vi "Send Message Immediate.vi"(8 "error in":errorcluster, 10 "IMessage":refnum<class "IMessage.lvclass">, 11 "Simulated CANopen Node in":refnum<class "Simulated CANopen Node.lvclass">) -> (0 "error out":errorcluster, 3 "Simulated CANopen Node out":refnum<class "Simulated CANopen Node.lvclass">)   [LabVIEW 2020, in "Simulated CANopen Node.lvclass"]
uses:
  Simulated CANopen Node.lvclass
  HAL/Source/Interfaces/IMessage/IMessage.lvclass
  Simulated CANopen Node.lvclass/Simulated CANopen Node.ctl
  HAL/Source/Messages/CAN CC Frame/CAN CC Frame.lvclass
  fe5fc66b-27c7-4b70-867a-ed015ee1e4a2.vi
  eee18dc1-6225-4693-ac9d-30609a8fa5c9.vi
  17ac248f-ac84-4826-aeec-a58701ccab40.vi
  98e92c24-c08f-4278-8538-098933e240cd.vi
  56a45396-c398-4984-a56f-735f0d2926b6.vi
  7e0a11d8-4694-4177-9e19-67e5199e02f7.vi
  5fa304e1-3e3d-4d0b-887e-d9a5c5a4f673.vi
  7c59c303-af64-4ebe-8db4-2588cd71c9a9.vi
  1c0038d2-8b70-42b8-b8fb-ff38a0514d58.vi
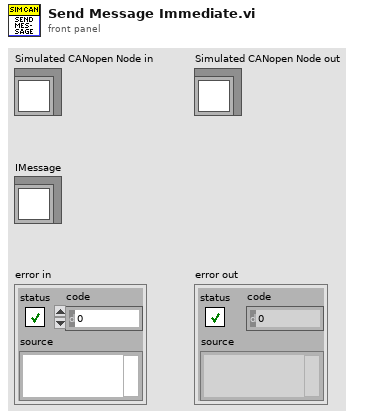
[diagram p1: front panel]
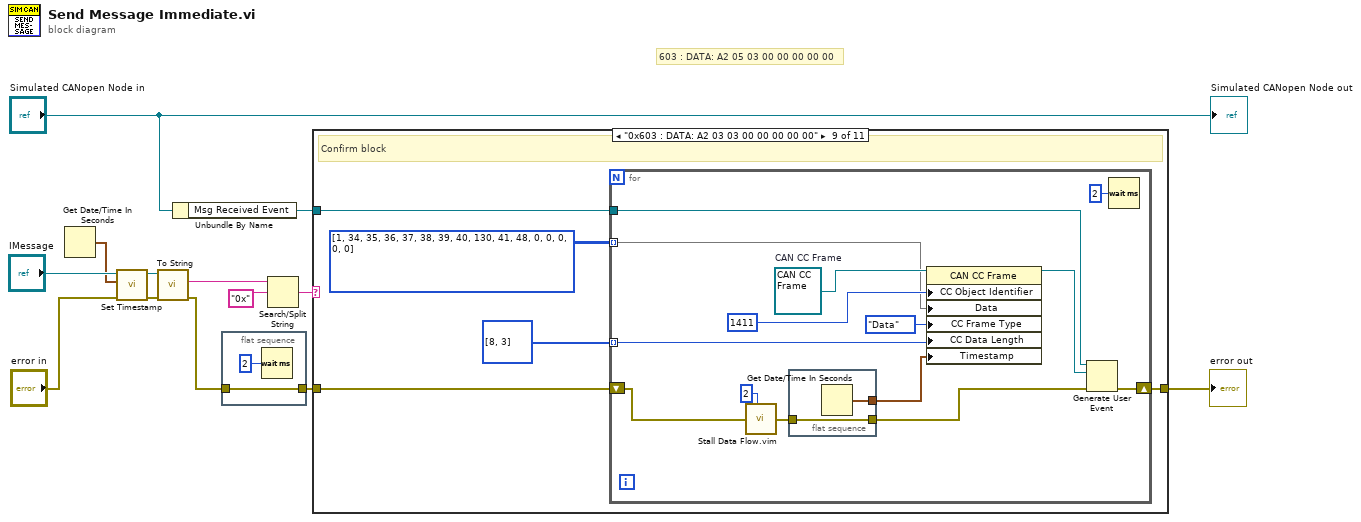
[diagram p0: block diagram]
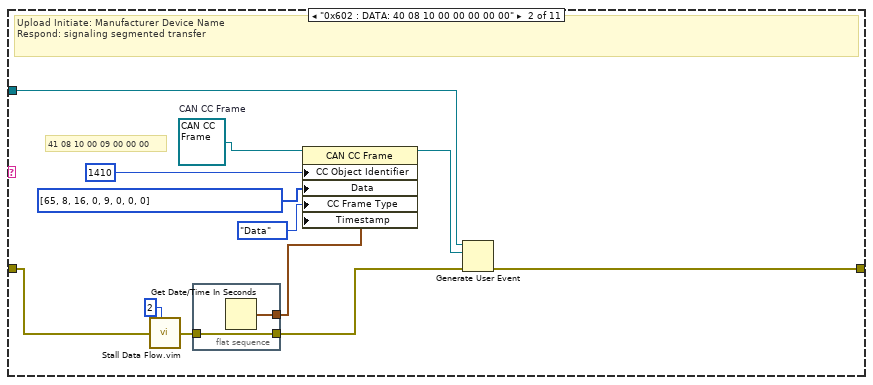
[diagram p3: hidden frame]
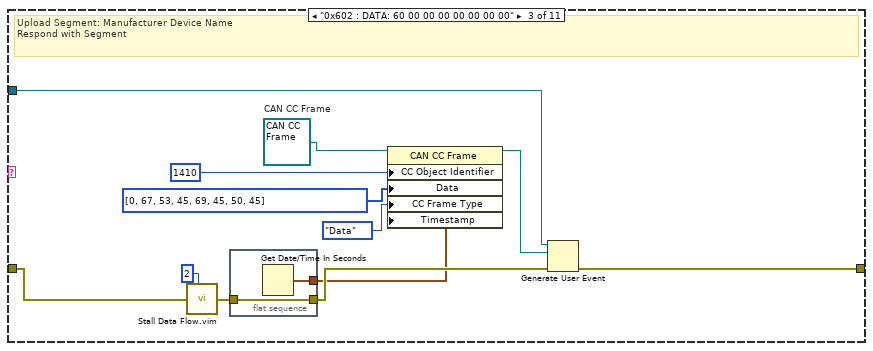
[diagram p4: hidden frame]
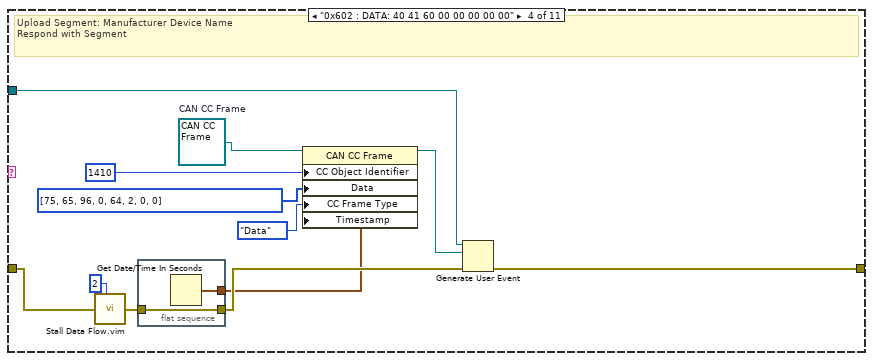
[diagram p5: hidden frame]
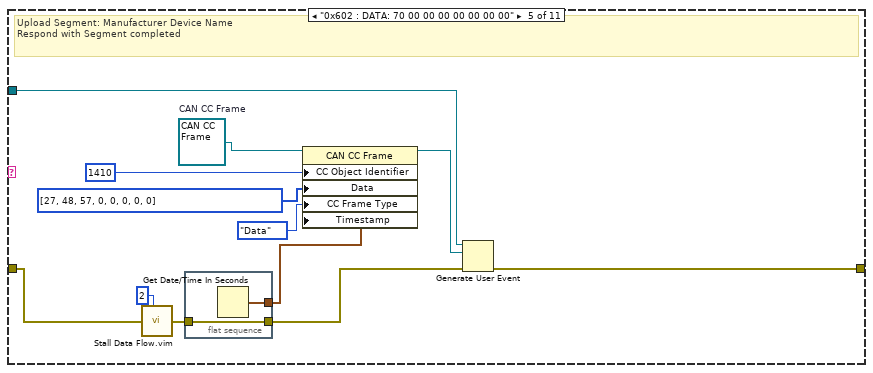
[diagram p6: hidden frame]
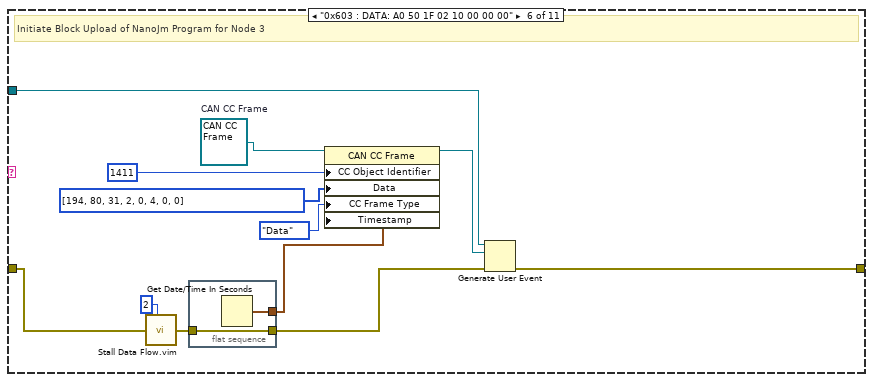
[diagram p7: hidden frame]
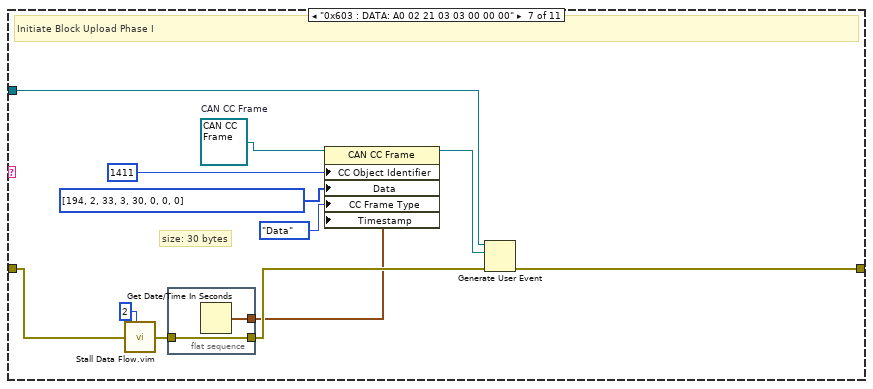
[diagram p8: hidden frame]
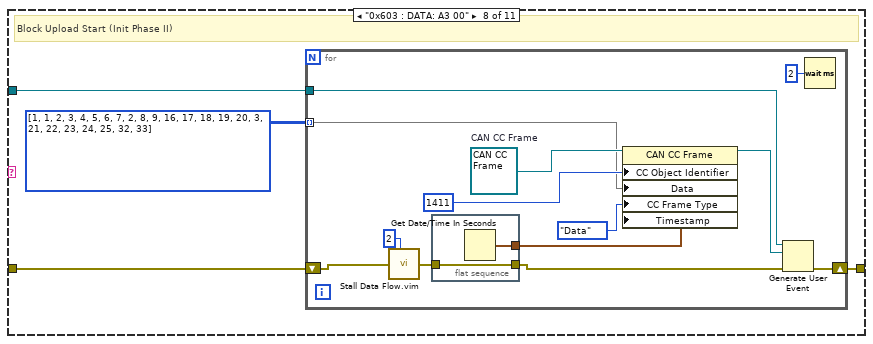
[diagram p9: hidden frame]
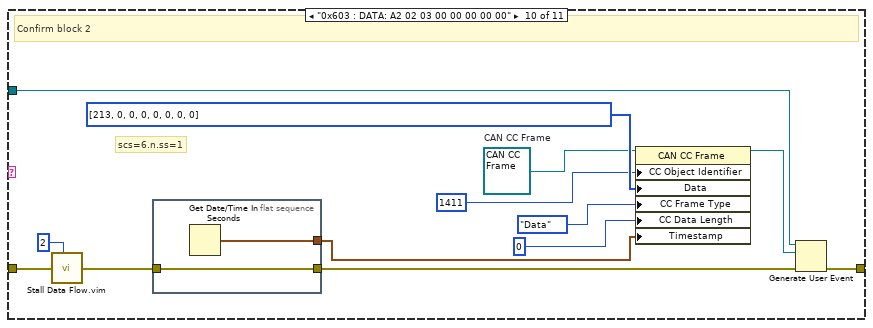
[diagram p10: hidden frame]
diagram:
  # "603 : DATA: A2 05 03 00 00 00 00 00"
  n1 = Get Date/Time In Seconds() -> (seconds since 1Jan1904=w1:timestamp)
  n2 = call-dynamic "Set Timestamp.vi"("error in"="error in", "Time Stamp"=w1, "IMessage in"="IMessage") -> ("error out"=w4:errorcluster, "IMessage out"=w2:refnum<class "IMessage.lvclass">)  [unwired: 7 in]
  n3 = call-dynamic "To String.vi"("error in"=w4, "IMessage in"=w2) -> ("error out"=w6:errorcluster, "Stringified"=w11:string)  [unwired: 7 in, 1 out]
  n4 = Unbundle By Name("Simulated CANopen Node in") -> ("Msg Received Event"=w9:refnum<user-event>)
  n5 = flat-sequence {
    tunnel: w6 -> [w14]
    tunnel: [w14] -> w5
    frame #0 {
      n6 = Wait (ms)(milliseconds to wait=u32 2) -> ()  [unwired: 1 out]
    }
  }
  n7 = Search/Split String(string=w11, search string/char (-)="0x") -> (match + rest of string=w7:string)  [unwired: 1 in, 2 out]
  n8 = case shown="\"0x603 : DATA: A2 03 03 00 00 00 00 00\"" w7 {
    tunnel: w5 -> [w16 w19 w33 w47 w61 w75 w89 w103 w120 w152 w156]
    tunnel: w9 -> [_ w24 w38 w52 w66 w78 w92 w101 w122 w150 _]
    tunnel: [w16 w22 w36 w50 w64 w79 w93 w102 w123 w151 w156] -> w8
    frame Default {
    }
    frame "0x602 : DATA: 40 08 10 00 00 00 00 00" {
      w28 = refnum<class "CAN CC Frame.lvclass"> refnum  # CAN CC Frame
      # "41 08 10 00 09 00 00 00"
      # "Upload Initiate: Manufacturer Device Name\nRespond: signaling segmented transfer"
      n9 = call "Stall Data Flow.vim"("value in"=w19, "milliseconds to wait"=u32 2) -> ("value out"=w20:errorcluster)  [unwired: 1 out]
      n10 = flat-sequence {
        tunnel: w20 -> [w30]
        tunnel: [w30] -> w18
        tunnel: [w29] -> w17
        frame #0 {
          n11 = Get Date/Time In Seconds() -> (seconds since 1Jan1904=w29:timestamp)
        }
      }
      n12 = property class="CAN CC Frame"(reference=w28, "CC Object Identifier"=u32 1410 ("COB-ID"), "Data"=u8[] [65, 8, 16, 0, 9, 0, 0, 0], "CC Frame Type"=enum8{"Data", "Remote", "Error", "Overload"}."Data", "Timestamp"=w17) -> (reference out=w23:refnum<class "CAN CC Frame.lvclass">)  [unwired: 1 in, 1 out]
      n13 = Generate User Event(user event=w24, event data cluster=w23, error in=w18) -> (error out=w22:errorcluster)  [unwired: 1 in, 1 out]
    }
    frame "0x602 : DATA: 60 00 00 00 00 00 00 00" {
      w42 = refnum<class "CAN CC Frame.lvclass"> refnum  # CAN CC Frame
      # "Upload Segment: Manufacturer Device Name\nRespond with Segment"
      n14 = call "Stall Data Flow.vim"("value in"=w33, "milliseconds to wait"=u32 2) -> ("value out"=w34:errorcluster)  [unwired: 1 out]
      n15 = flat-sequence {
        tunnel: w34 -> [w44]
        tunnel: [w44] -> w32
        tunnel: [w43] -> w31
        frame #0 {
          n16 = Get Date/Time In Seconds() -> (seconds since 1Jan1904=w43:timestamp)
        }
      }
      n17 = property class="CAN CC Frame"(reference=w42, "CC Object Identifier"=u32 1410 ("COB-ID"), "Data"=u8[] [0, 67, 53, 45, 69, 45, 50, 45], "CC Frame Type"=enum8{"Data", "Remote", "Error", "Overload"}."Data", "Timestamp"=w31) -> (reference out=w37:refnum<class "CAN CC Frame.lvclass">)  [unwired: 1 in, 1 out]
      n18 = Generate User Event(user event=w38, event data cluster=w37, error in=w32) -> (error out=w36:errorcluster)  [unwired: 1 in, 1 out]
    }
    frame "0x602 : DATA: 40 41 60 00 00 00 00 00" {
      w56 = refnum<class "CAN CC Frame.lvclass"> refnum  # CAN CC Frame
      # "Upload Segment: Manufacturer Device Name\nRespond with Segment"
      n19 = call "Stall Data Flow.vim"("value in"=w47, "milliseconds to wait"=u32 2) -> ("value out"=w48:errorcluster)  [unwired: 1 out]
      n20 = flat-sequence {
        tunnel: w48 -> [w58]
        tunnel: [w58] -> w46
        tunnel: [w57] -> w45
        frame #0 {
          n21 = Get Date/Time In Seconds() -> (seconds since 1Jan1904=w57:timestamp)
        }
      }
      n22 = property class="CAN CC Frame"(reference=w56, "CC Object Identifier"=u32 1410 ("COB-ID"), "Data"=u8[] [75, 65, 96, 0, 64, 2, 0, 0], "CC Frame Type"=enum8{"Data", "Remote", "Error", "Overload"}."Data", "Timestamp"=w45) -> (reference out=w51:refnum<class "CAN CC Frame.lvclass">)  [unwired: 1 in, 1 out]
      n23 = Generate User Event(user event=w52, event data cluster=w51, error in=w46) -> (error out=w50:errorcluster)  [unwired: 1 in, 1 out]
    }
    frame "0x602 : DATA: 70 00 00 00 00 00 00 00" {
      w70 = refnum<class "CAN CC Frame.lvclass"> refnum  # CAN CC Frame
      # "Upload Segment: Manufacturer Device Name\nRespond with Segment completed"
      n24 = call "Stall Data Flow.vim"("value in"=w61, "milliseconds to wait"=u32 2) -> ("value out"=w62:errorcluster)  [unwired: 1 out]
      n25 = flat-sequence {
        tunnel: w62 -> [w72]
        tunnel: [w72] -> w60
        tunnel: [w71] -> w59
        frame #0 {
          n26 = Get Date/Time In Seconds() -> (seconds since 1Jan1904=w71:timestamp)
        }
      }
      n27 = property class="CAN CC Frame"(reference=w70, "CC Object Identifier"=u32 1410 ("COB-ID"), "Data"=u8[] [27, 48, 57, 0, 0, 0, 0, 0], "CC Frame Type"=enum8{"Data", "Remote", "Error", "Overload"}."Data", "Timestamp"=w59) -> (reference out=w65:refnum<class "CAN CC Frame.lvclass">)  [unwired: 1 in, 1 out]
      n28 = Generate User Event(user event=w66, event data cluster=w65, error in=w60) -> (error out=w64:errorcluster)  [unwired: 1 in, 1 out]
    }
    frame "0x603 : DATA: A0 50 1F 02 10 00 00 00" {
      w84 = refnum<class "CAN CC Frame.lvclass"> refnum  # CAN CC Frame
      # "Initiate Block Upload of NanoJm Program for Node 3"
      n29 = call "Stall Data Flow.vim"("value in"=w75, "milliseconds to wait"=u32 2) -> ("value out"=w76:errorcluster)  [unwired: 1 out]
      n30 = flat-sequence {
        tunnel: w76 -> [w86]
        tunnel: [w86] -> w74
        tunnel: [w85] -> w73
        frame #0 {
          n31 = Get Date/Time In Seconds() -> (seconds since 1Jan1904=w85:timestamp)
        }
      }
      n32 = property class="CAN CC Frame"(reference=w84, "CC Object Identifier"=u32 1411 ("COB-ID"), "Data"=u8[] [194, 80, 31, 2, 0, 4, 0, 0], "CC Frame Type"=enum8{"Data", "Remote", "Error", "Overload"}."Data", "Timestamp"=w73) -> (reference out=w80:refnum<class "CAN CC Frame.lvclass">)  [unwired: 1 in, 1 out]
      n33 = Generate User Event(user event=w78, event data cluster=w80, error in=w74) -> (error out=w79:errorcluster)  [unwired: 1 in, 1 out]
    }
    frame "0x603 : DATA: A0 02 21 03 03 00 00 00" {
      w98 = refnum<class "CAN CC Frame.lvclass"> refnum  # CAN CC Frame
      # "size: 30 bytes"
      # "Initiate Block Upload Phase I"
      n34 = call "Stall Data Flow.vim"("value in"=w89, "milliseconds to wait"=u32 2) -> ("value out"=w90:errorcluster)  [unwired: 1 out]
      n35 = flat-sequence {
        tunnel: w90 -> [w100]
        tunnel: [w100] -> w88
        tunnel: [w99] -> w87
        frame #0 {
          n36 = Get Date/Time In Seconds() -> (seconds since 1Jan1904=w99:timestamp)
        }
      }
      n37 = property class="CAN CC Frame"(reference=w98, "CC Object Identifier"=u32 1411 ("COB-ID"), "Data"=u8[] [194, 2, 33, 3, 30, 0, 0, 0], "CC Frame Type"=enum8{"Data", "Remote", "Error", "Overload"}."Data", "Timestamp"=w87) -> (reference out=w94:refnum<class "CAN CC Frame.lvclass">)  [unwired: 1 in, 1 out]
      n38 = Generate User Event(user event=w92, event data cluster=w94, error in=w88) -> (error out=w93:errorcluster)  [unwired: 1 in, 1 out]
    }
    frame "0x603 : DATA: A3 00" {
      # "Block Upload Start (Init Phase II)"
      n39 = for {
        tunnel: u8[][] [[1, 1, 2, 3, 4, 5, 6, 7], [2, 8, 9, 16, 17, 18, 19, 20], [3, 21, 22, 23, 24, 25, 32, 33]] ("Data") -> [w115] mode=indexing
        tunnel: w101 -> [w111]
        shift-right: [w112] -> w102
        shift-left: w103 -> [w107]
        w117 = refnum<class "CAN CC Frame.lvclass"> refnum  # CAN CC Frame
        n40 = call "Stall Data Flow.vim"("value in"=w107, "milliseconds to wait"=u32 2) -> ("value out"=w108:errorcluster)  [unwired: 1 out]
        n41 = flat-sequence {
          tunnel: w108 -> [w119]
          tunnel: [w119] -> w106
          tunnel: [w118] -> w105
          frame #0 {
            n42 = Get Date/Time In Seconds() -> (seconds since 1Jan1904=w118:timestamp)
          }
        }
        n43 = property class="CAN CC Frame"(reference=w117, "CC Object Identifier"=u32 1411 ("COB-ID"), "Data"=w115, "CC Frame Type"=enum8{"Data", "Remote", "Error", "Overload"}."Data", "Timestamp"=w105) -> (reference out=w113:refnum<class "CAN CC Frame.lvclass">)  [unwired: 1 in, 1 out]
        n44 = Generate User Event(user event=w111, event data cluster=w113, error in=w106) -> (error out=w112:errorcluster)  [unwired: 1 in, 1 out]
        n45 = Wait (ms)(milliseconds to wait=u32 2) -> ()  [unwired: 1 out]
      }
    }
    frame "0x603 : DATA: A2 03 03 00 00 00 00 00" {
      # "Confirm block"
      n46 = for {
        tunnel: u8[][] [[1, 34, 35, 36, 37, 38, 39, 40], [130, 41, 48, 0, 0, 0, 0, 0]] ("Data") -> [w136] mode=indexing
        tunnel: w122 -> [w132]
        shift-right: [w133] -> w123
        shift-left: w120 -> [w127]
        tunnel: u8[] [8, 3] -> [w130] mode=indexing
        w138 = refnum<class "CAN CC Frame.lvclass"> refnum  # CAN CC Frame
        n47 = call "Stall Data Flow.vim"("value in"=w127, "milliseconds to wait"=u32 2) -> ("value out"=w128:errorcluster)  [unwired: 1 out]
        n48 = flat-sequence {
          tunnel: w128 -> [w140]
          tunnel: [w140] -> w126
          tunnel: [w139] -> w125
          frame #0 {
            n49 = Get Date/Time In Seconds() -> (seconds since 1Jan1904=w139:timestamp)
          }
        }
        n50 = property class="CAN CC Frame"(reference=w138, "CC Object Identifier"=u32 1411 ("COB-ID"), "Data"=w136, "CC Frame Type"=enum8{"Data", "Remote", "Error", "Overload"}."Data", "CC Data Length"=w130, "Timestamp"=w125) -> (reference out=w134:refnum<class "CAN CC Frame.lvclass">)  [unwired: 1 in, 1 out]
        n51 = Generate User Event(user event=w132, event data cluster=w134, error in=w126) -> (error out=w133:errorcluster)  [unwired: 1 in, 1 out]
        n52 = Wait (ms)(milliseconds to wait=u32 2) -> ()  [unwired: 1 out]
      }
    }
    frame "0x603 : DATA: A2 02 03 00 00 00 00 00" {
      w149 = refnum<class "CAN CC Frame.lvclass"> refnum  # CAN CC Frame
      # "scs=6.n.ss=1"
      # "Confirm block 2"
      n53 = call "Stall Data Flow.vim"("value in"=w152, "milliseconds to wait"=u32 2) -> ("value out"=w143:errorcluster)  [unwired: 1 out]
      n54 = flat-sequence {
        tunnel: w143 -> [w155]
        tunnel: [w155] -> w142
        tunnel: [w154] -> w141
        frame #0 {
          n55 = Get Date/Time In Seconds() -> (seconds since 1Jan1904=w154:timestamp)
        }
      }
      n56 = property class="CAN CC Frame"(reference=w149, "CC Object Identifier"=u32 1411 ("COB-ID"), "Data"=u8[] [213, 0, 0, 0, 0, 0, 0, 0], "CC Frame Type"=enum8{"Data", "Remote", "Error", "Overload"}."Data", "CC Data Length"=u8 0, "Timestamp"=w141) -> (reference out=w146:refnum<class "CAN CC Frame.lvclass">)  [unwired: 1 in, 1 out]
      n57 = Generate User Event(user event=w150, event data cluster=w146, error in=w142) -> (error out=w151:errorcluster)  [unwired: 1 in, 1 out]
    }
    frame "0x603 : DATA: A1 00 00 00 00 00 00" {
      # "End block resp"
    }
  }
  "error out" <- w8
  "Simulated CANopen Node out" <- "Simulated CANopen Node in"
